vi "动态图.vi"() -> ()   [LabVIEW 2016, in "PLC.lvlib"]
uses:
  PLC.lvlib
  C:/Program Files (x86)/National Instruments/LabVIEW 2016/examples/lvdsc/XControls/Animator/Control/AnimatorXControl.xctl
panel:
  in  "Mixer speed":dbl(knob)=8.0 scale=0.0..25.0
  in  "AnimatorXControl-Mixer":u32(xcontrol)
  in  "Flow speed":dbl(knob)=5.0 scale=0.0..25.0
  in  "stop":bool
  in  "AnimatorXControl-Flow":u32(xcontrol)
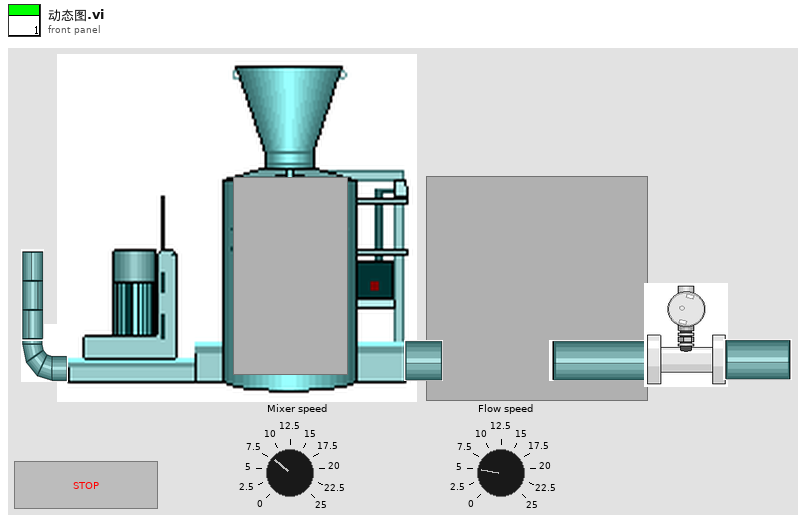
[diagram p1: front panel]
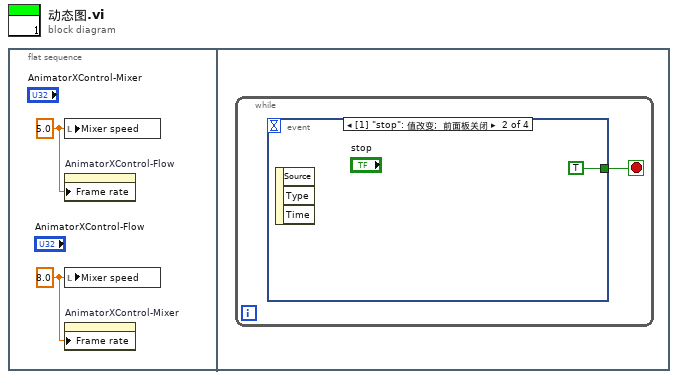
[diagram p0: block diagram]
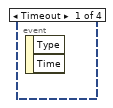
[diagram p2: hidden frame]
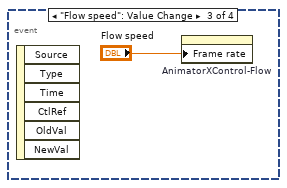
[diagram p3: hidden frame]
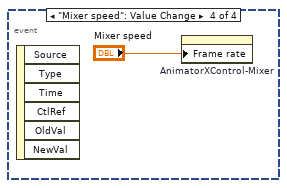
[diagram p4: hidden frame]
diagram:
  n1 = flat-sequence {
    frame #0 {
      w1 = 5.0 ("Speed 2")
      w2 = 8.0 ("Speed 1")
      n2 = local write "Mixer speed"(w1) -> ()
      n3 = property on="AnimatorXControl-Flow" class="AnimatorXControl (严格)"("Frame rate"=w1) -> ()  [unwired: 2 in, 2 out]
      n4 = local write "Mixer speed"(w2) -> ()
      n5 = property on="AnimatorXControl-Mixer" class="AnimatorXControl (严格)"("Frame rate"=w2) -> ()  [unwired: 2 in, 2 out]
    }
    frame #1 {
      n6 = while {
        stop <- w3 stop-if-true
        n7 = event shown="[1] \"stop\": 值改变;  前面板关闭" {
          selector: _ -> [_ _ _ _]
          dyn-events: _ -> [_ _ _ _]
          timeout: _ -> [_ _ _ _]
          tunnel: [_ TRUE _ _] -> w3
          event Timeout {
            n8 = event-data() -> ()  [unwired: 1 in, 2 out]
          }
          event "stop": Value Change; Panel Close {
            n9 = event-data() -> ()  [unwired: 1 in, 3 out]
          }
          event "Flow speed": Value Change {
            n10 = event-data() -> ()  [unwired: 1 in, 6 out]
            n11 = property on="AnimatorXControl-Flow" class="AnimatorXControl (严格)"("Frame rate"="Flow speed") -> ()  [unwired: 2 in, 2 out]
          }
          event "Mixer speed": Value Change {
            n12 = event-data() -> ()  [unwired: 1 in, 6 out]
            n13 = property on="AnimatorXControl-Mixer" class="AnimatorXControl (严格)"("Frame rate"="Mixer speed") -> ()  [unwired: 2 in, 2 out]
          }
        }
      }
    }
  }
